vi "err2table.vi"(5 "err_table":string[](array[string]), 7 "Tbl Refnum":refnum<vi>) -> ()   [LabVIEW 2010]
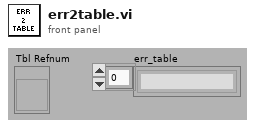
[diagram p1: front panel]
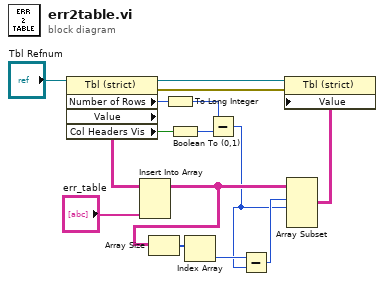
[diagram p0: block diagram]
diagram:
  n1 = property on="Property Node" class="Tbl (strict)"(reference="Tbl Refnum") -> (reference out=w7:refnum<vi>, error out=w6:errorcluster, "Number of Rows"=w4:u32, "Value"=w12:string[][], "Col Headers Vis"=w5:bool)  [unwired: 1 in]
  n2 = Insert Into Array(array=w12, new element="err_table") -> (w15:string[][])  [unwired: 2 in]
  n3 = Array Size(array=w15) -> (size(s)=w11:i32[])
  n4 = To Long Integer(number=w4) -> (32bit integer=w1:i32)
  n5 = Boolean To (0,1)(Boolean=w5) -> (0, 1=w3:i16)
  n6 = Index Array(array=w11) -> (element=w14:i32)  [unwired: 1 in]
  n7 = Subtract(x=w1, y=w3) -> (x-y=w2:i32)
  n8 = Subtract(x=w14, y=w2) -> (x-y=w13:i32)
  n9 = Array Subset(array=w15, index (row)=w13, length (row)=w2) -> (w9:string[][])  [unwired: 2 in]
  n10 = property on="Property Node" class="Tbl (strict)"(reference=w7, error in=w6, "Value"=w9) -> ()  [unwired: 2 out]
